vi "PicoScope3000aGetBlock.vi"(0 "error in":errorcluster, 2 "handle in":i16, 3 "Acquisition Settings":T4 {"Down Sample Ratio" min=1 step=1; "Down-Sample Mode" items=["None", "Aggregate", "Decimate", "Average"]}, 8 "Device Info":T1) -> (4 "overflow":i16, 5 "noOfSamples":u32, 6 "error out":errorcluster, 7 "handle out":i16, 9 "Buffers (Max or non-aggregated)":T3, 10 "Min Buffers":T2)   [LabVIEW 2009]
doc: "This VI collects a block of data from the oscilloscope. This can be called in a loop in order to continually collect blocks of data. The oscilloscope should first be set up by using PicoScope3000aSettings.vi. The VI outputs data arrays in two clusters (max and min). If not using aggregation, 'Min Buffers' is not used."
uses:
  ps3000a.dll
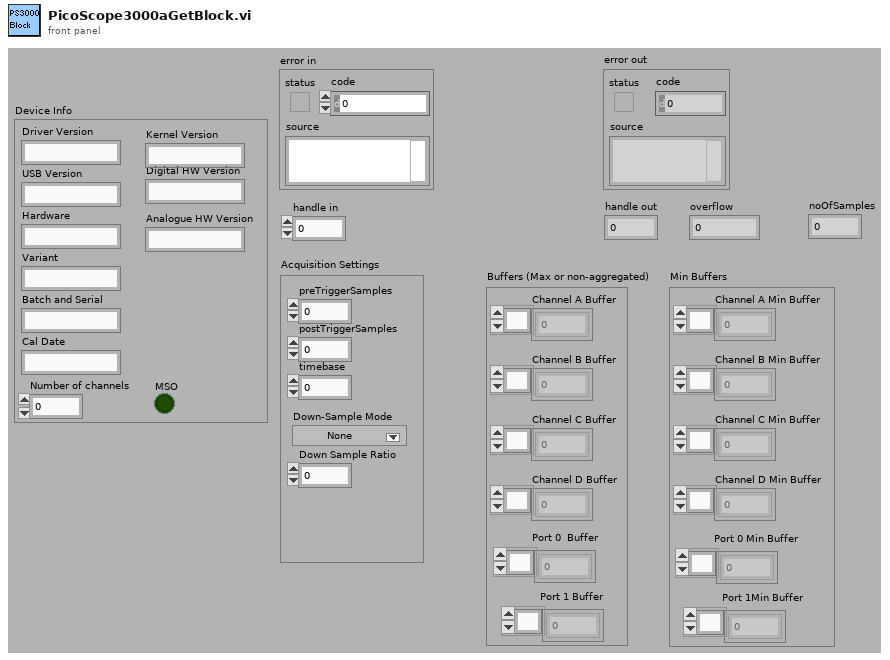
[diagram p1: front panel]
types:
  T1 = cluster{"Driver Version":string, "USB Version":string, "Hardware":string, "Variant":string, "Batch and Serial":string, "Cal Date":string, "Kernel Version":string, "Digital HW Version":string, "Analogue HW Version":string, "MSO":bool, "Number of channels":i16}
  T2 = cluster{"Channel A Min Buffer":i16[], "Channel B Min Buffer":i16[], "Channel C Min Buffer":i16[], "Channel D Min Buffer":i16[], "Port 0 Min Buffer ":i16[], "Port 1Min Buffer ":i16[]}
  T3 = cluster{"Channel D Buffer":i16[], "Channel C Buffer":i16[], "Channel B Buffer":i16[], "Channel A Buffer":i16[], "Port 0  Buffer ":i16[], "Port 1 Buffer ":i16[]}
  T4 = cluster{"preTriggerSamples":u32, "postTriggerSamples":u32, "timebase":u32, "Down-Sample Mode":i32, "Down Sample Ratio":u32}
  T5 = cluster{"Channel A Min Buffer":i16[], "Channel B Min Buffer":i16[], "Channel C Min Buffer":i16[], "Channel D Min Buffer":i16[], "Port 0 Min Buffer":i32[], "Port 1 Min Buffer":i32[]}
  T6 = cluster{"Channel D Buffer":i16[], "Channel C Buffer":i16[], "Channel B Buffer":i16[], "Channel A Buffer":i16[], "Port 0 Max Buffer":i32[], "Port 1 Max Buffer":i32[]}
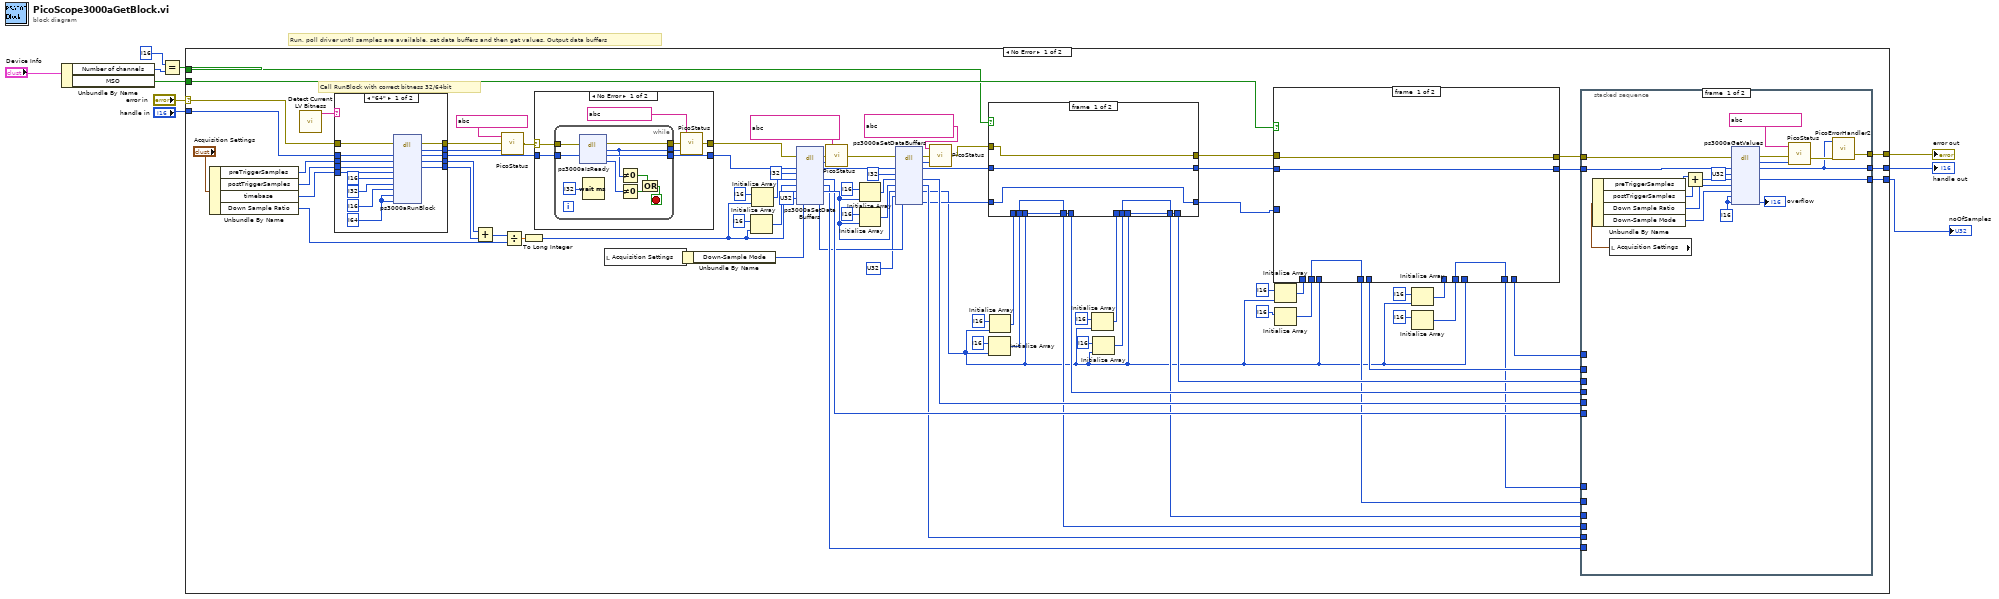
[diagram p0: block diagram]
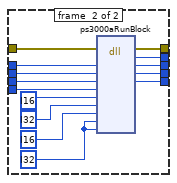
[diagram p2: hidden frame]
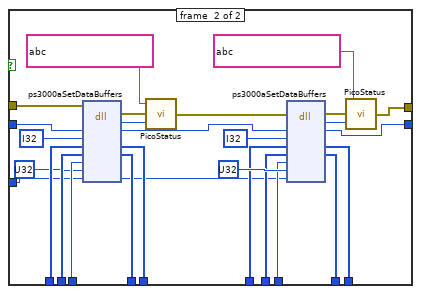
[diagram p3: hidden frame]
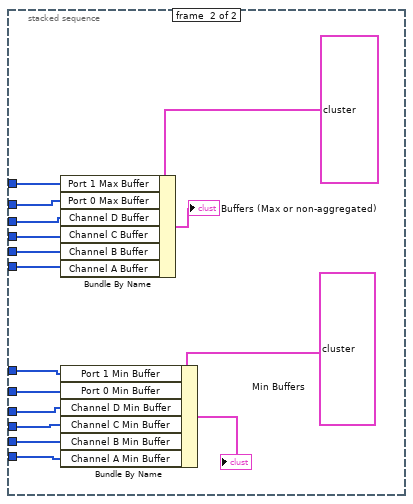
[diagram p4: hidden frame]
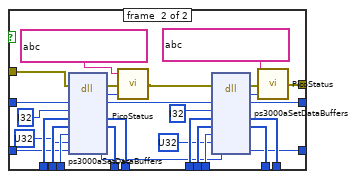
[diagram p6: hidden frame]
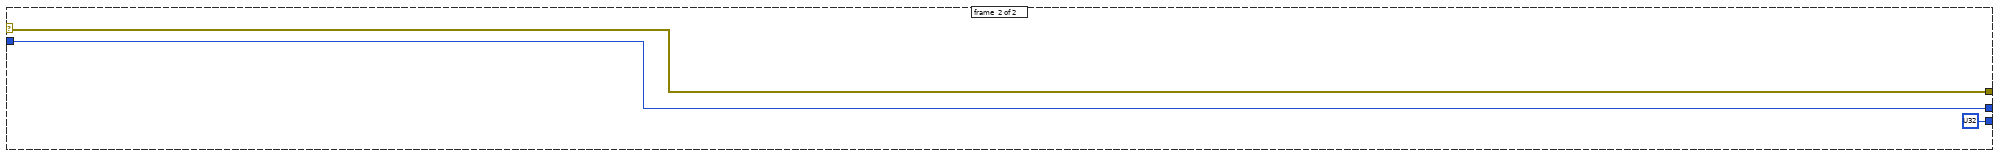
[diagram p7: hidden frame]
diagram:
  # "Run, poll driver until samples are available, set data buffers and then get values. Output data buffers"
  n1 = Unbundle By Name("Device Info") -> ("Number of channels"=w4:i16, "MSO"=w3:bool)
  n2 = Equal?(x=i16 ?, y=w4) -> (x = y?=w2:bool)
  n3 = case shown="No Error" "error in" {
    selector: "error in" -> [w64 w248]
    tunnel: [w65 w248] -> w9
    tunnel: "handle in" -> [w63 w247]
    tunnel: [w62 w247] -> w7
    tunnel: [w15 u32 ? ("noOfSamples")] -> w6
    tunnel: w3 -> [w13 _]
    tunnel: w2 -> [w12 _]
    frame #0 {
      # "Call RunBlock with correct bitness 32/64bit"
      n4 = Unbundle By Name("Acquisition Settings") -> ("preTriggerSamples"=w79:u32, "postTriggerSamples"=w78:u32, "timebase"=w80:u32, "Down Sample Ratio"=w14:u32)
      n5 = call "Detect Current LV Bitness.vi"() -> ("bitness"=w11:string)  [unwired: 11 in]
      n6 = case shown="\"64\"" w11 {
        tunnel: [w110 w124] -> w96
        tunnel: [w109 w123] -> w92
        tunnel: [w108 w122] -> w91
        tunnel: w80 -> [w107 w121]
        tunnel: w79 -> [w106 w120]
        tunnel: w78 -> [w105 w119]
        tunnel: [w104 w118] -> w77
        tunnel: [w103 w117] -> w76
        tunnel: w64 -> [w102 w116]
        tunnel: w63 -> [w101 w115]
        frame #0 {
          w97 = i64 ? ("pParameter")
          n7 = dll-call lib="ps3000a.dll" fn="ps3000aRunBlock" ("ps3000.dll:_ps3000_open_unit@0")(error in=w102, "handle"=w101, "preTriggerSamples"=w106, "postTriggerSamples"=w105, "timebase"=w107, "oversample"=i16 ?, "timeindisposed"=i32 ? ("pParameter"), "segmentIndex"=i16 ? ("pParameter"), "lpReady"=w97, "pParameter"=w97) -> (error out=w103:errorcluster, "PICO_STATUS"=w104:i32, "handle"=w110:i16, "preTriggerSamples"=w109:u32, "postTriggerSamples"=w108:u32)  [unwired: 8 in, 1 out]
        }
        frame #1 {
          w111 = i32 ? ("pParameter")
          n8 = dll-call lib="ps3000a.dll" fn="ps3000aRunBlock" ("ps3000.dll:_ps3000_open_unit@0")(error in=w116, "handle"=w115, "preTriggerSamples"=w120, "postTriggerSamples"=w119, "timebase"=w121, "oversample"=i16 ?, "timeindisposed"=i32 ? ("pParameter"), "segmentIndex"=i16 ? ("pParameter"), "lpReady"=w111, "pParameter"=w111) -> (error out=w117:errorcluster, "PICO_STATUS"=w118:i32, "handle"=w124:i16, "preTriggerSamples"=w123:u32, "postTriggerSamples"=w122:u32)  [unwired: 8 in, 1 out]
        }
      }
      n9 = Add(x=w92, y=w91) -> (x+y=w42:u32)
      n10 = call "PicoStatus.vi"("PICO STATUS"=w77, "error in"=w76, "source"=string ?) -> ("error out"=w75:errorcluster)
      n11 = Divide(x=w42, y=w14) -> (x/y=w41:dbl)
      n12 = To Long Integer(number=w41) -> (32bit integer=w40:i32)
      n13 = case shown="No Error" w75 {
        selector: w75 -> [w195 w208]
        tunnel: w96 -> [w197 w209]
        tunnel: [w196 w209] -> w95
        tunnel: [w194 w208] -> w83
        frame #0 {
          n14 = while {
            tunnel: [w207] -> w196
            tunnel: w197 -> [w206]
            tunnel: [w201] -> w192
            tunnel: w195 -> [w200]
            tunnel: [w199] -> w193
            stop <- w205 stop-if-true
            n15 = dll-call lib="ps3000a.dll" fn="ps3000aIsReady" ("ps3000.dll:_ps3000_open_unit@0")(error in=w200, "handle"=w206) -> (error out=w199:errorcluster, "status"=w201:i32, "handle"=w207:i16, "ready"=w202:i16)  [unwired: 3 in, 1 out]
            n16 = Wait (ms)(milliseconds to wait=i32 ?) -> ()  [unwired: 1 out]
            n17 = Not Equal To 0?(x=w201) -> (x != 0?=w203:bool)
            n18 = Not Equal To 0?(x=w202) -> (x != 0?=w204:bool)
            n19 = Or(x=w203, y=w204) -> (x .or. y?=w205:bool)
          }
          n20 = call "PicoStatus.vi"("PICO STATUS"=w192, "error in"=w193, "source"=string ?) -> ("error out"=w194:errorcluster)
        }
        frame #1 {
        }
      }
      n21 = local read "Acquisition Settings"() -> (w39:T4)
      n22 = Unbundle By Name(w39) -> ("Down-Sample Mode"=w37:i32)
      n23 = Initialize Array(i16 ? ("element"), w40) -> (w60:i16[])
      n24 = Initialize Array(i16 ? ("element"), w40) -> (w90:i16[])
      n25 = dll-call lib="ps3000a.dll" fn="ps3000aSetDataBuffers" ("ps3000.dll:_ps3000_open_unit@0")(error in=w83, "handle"=w95, "channel"=i32 ?, "bufferMax"=w90, "bufferMin"=w60, "bufferLth"=w40, "segmentIndex"=u32 ?, "mode"=w37) -> (error out=w73:errorcluster, "PICO_STATUS"=w74:i32, "handle"=w94:i16, "bufferMax"=w47:i16[], "bufferMin"=w43:i16[], "bufferLth"=w51:i32, "mode"=w36:i32)  [unwired: 4 in, 1 out]
      n26 = call "PicoStatus.vi"("PICO STATUS"=w74, "error in"=w73, "source"=string ?) -> ("error out"=w72:errorcluster)
      n27 = Initialize Array(i16 ? ("element"), w51) -> (w87:i16[])
      n28 = Initialize Array(i16 ? ("element"), w51) -> (w58:i16[])
      n29 = dll-call lib="ps3000a.dll" fn="ps3000aSetDataBuffers" ("ps3000.dll:_ps3000_open_unit@0")(error in=w72, "handle"=w94, "channel"=i32 ?, "bufferMax"=w87, "bufferMin"=w58, "bufferLth"=w51, "segmentIndex"=u32 ?, "mode"=w36) -> (error out=w70:errorcluster, "PICO_STATUS"=w71:i32, "handle"=w93:i16, "bufferMax"=w48:i16[], "bufferMin"=w44:i16[], "bufferLth"=w16:i32, "mode"=w35:i32)  [unwired: 4 in, 1 out]
      n30 = call "PicoStatus.vi"("PICO STATUS"=w71, "error in"=w70, "source"=string ?) -> ("error out"=w69:errorcluster)
      n31 = Initialize Array(i16 ? ("element"), w16) -> (w55:i16[])
      n32 = Initialize Array(i16 ? ("element"), w16) -> (w86:i16[])
      n33 = Initialize Array(i16 ? ("element"), w16) -> (w85:i16[])
      n34 = Initialize Array(i16 ? ("element"), w16) -> (w52:i16[])
      n35 = case shown="True" w12 {
        tunnel: w93 -> [w214 w245]
        tunnel: [w214 w243] -> w24
        tunnel: w86 -> [w216 w242]
        tunnel: w85 -> [w215 w241]
        tunnel: [w215 w240] -> w50
        tunnel: [w216 w239] -> w49
        tunnel: w69 -> [w213 w236]
        tunnel: [w213 w230] -> w25
        tunnel: w55 -> [w212 w227]
        tunnel: w52 -> [w211 w226]
        tunnel: [w211 w225] -> w46
        tunnel: [w212 w224] -> w45
        tunnel: w16 -> [_ w223]
        tunnel: w16 -> [_ w222]
        tunnel: w35 -> [w210 w221]
        tunnel: [w210 w217] -> w21
        frame #0 {
        }
        frame #1 {
          n36 = dll-call lib="ps3000a.dll" fn="ps3000aSetDataBuffers" ("ps3000.dll:_ps3000_open_unit@0")(error in=w236, "handle"=w245, "channel"=i32 ?, "bufferMax"=w242, "bufferMin"=w227, "bufferLth"=w223, "segmentIndex"=u32 ?, "mode"=w221) -> (error out=w234:errorcluster, "PICO_STATUS"=w235:i32, "handle"=w244:i16, "bufferMax"=w239:i16[], "bufferMin"=w224:i16[], "mode"=w220:i32)  [unwired: 5 in, 1 out]
          n37 = call "PicoStatus.vi"("PICO STATUS"=w235, "error in"=w234, "source"=string ?) -> ("error out"=w233:errorcluster)
          n38 = dll-call lib="ps3000a.dll" fn="ps3000aSetDataBuffers" ("ps3000.dll:_ps3000_open_unit@0")(error in=w233, "handle"=w244, "channel"=i32 ?, "bufferMax"=w241, "bufferMin"=w226, "bufferLth"=w222, "segmentIndex"=u32 ?, "mode"=w220) -> (error out=w231:errorcluster, "PICO_STATUS"=w232:i32, "handle"=w243:i16, "bufferMax"=w240:i16[], "bufferMin"=w225:i16[], "mode"=w217:i32)  [unwired: 5 in, 1 out]
          n39 = call "PicoStatus.vi"("PICO STATUS"=w232, "error in"=w231, "source"=string ?) -> ("error out"=w230:errorcluster)
        }
      }
      n40 = Initialize Array(i16 ? ("element"), w16) -> (w31:i16[])
      n41 = Initialize Array(i16 ? ("element")) -> (w30:i16[])  [unwired: 1 in]
      n42 = Initialize Array(i16 ? ("element"), w16) -> (w26:i16[])
      n43 = Initialize Array(i16 ? ("element")) -> (w27:i16[])  [unwired: 1 in]
      n44 = case shown="True" w13 {
        tunnel: w25 -> [w126 w156]
        tunnel: w24 -> [w125 w155]
        tunnel: w31 -> [_ w153]
        tunnel: w30 -> [w128 w152]
        tunnel: w16 -> [_ w151]
        tunnel: w16 -> [_ w145]
        tunnel: w27 -> [w127 w146]
        tunnel: w26 -> [_ w147]
        tunnel: [w128 w144] -> w17
        tunnel: [_ w143] -> w19
        tunnel: [w127 w142] -> w18
        tunnel: [_ w141] -> w20
        tunnel: [w125 w135] -> w22
        tunnel: [w126 w134] -> w23
        tunnel: w21 -> [_ w132]
        frame #0 {
        }
        frame #1 {
          n45 = dll-call lib="ps3000a.dll" fn="ps3000aSetDataBuffers" ("ps3000.dll:_ps3000_open_unit@0")(error in=w156, "handle"=w155, "channel"=i32 ?, "bufferMax"=w153, "bufferMin"=w152, "bufferLth"=w151, "segmentIndex"=u32 ?, "mode"=w132) -> (error out=w139:errorcluster, "PICO_STATUS"=w140:i32, "handle"=w133:i16, "bufferMax"=w143:i16[], "bufferMin"=w144:i16[], "mode"=w131:i32)  [unwired: 5 in, 1 out]
          n46 = call "PicoStatus.vi"("PICO STATUS"=w140, "error in"=w139, "source"=string ?) -> ("error out"=w136:errorcluster)
          n47 = dll-call lib="ps3000a.dll" fn="ps3000aSetDataBuffers" ("ps3000.dll:_ps3000_open_unit@0")(error in=w136, "handle"=w133, "channel"=i32 ?, "bufferMax"=w147, "bufferMin"=w146, "bufferLth"=w145, "segmentIndex"=u32 ?, "mode"=w131) -> (error out=w137:errorcluster, "PICO_STATUS"=w138:i32, "handle"=w135:i16, "bufferMax"=w141:i16[], "bufferMin"=w142:i16[])  [unwired: 6 in, 1 out]
          n48 = call "PicoStatus.vi"("PICO STATUS"=w138, "error in"=w137, "source"=string ?) -> ("error out"=w134:errorcluster)
        }
      }
      n49 = stacked-sequence {
        tunnel: w22 -> [w174 _]
        tunnel: [w168 _] -> w65
        tunnel: [w157 _] -> w62
        tunnel: w50 -> [_ w180]
        tunnel: w49 -> [_ w181]
        tunnel: w48 -> [_ w182]
        tunnel: w47 -> [_ w179]
        tunnel: w46 -> [_ w186]
        tunnel: w45 -> [_ w185]
        tunnel: w44 -> [_ w184]
        tunnel: w43 -> [_ w183]
        tunnel: w23 -> [w160 _]
        tunnel: w20 -> [_ w178]
        tunnel: w19 -> [_ w177]
        tunnel: w18 -> [_ w176]
        tunnel: w17 -> [_ w175]
        tunnel: [w159 _] -> w15
        frame #0 {
          w172 = i16 ? ("overflow")
          n50 = local read "Acquisition Settings"() -> (w166:T4)
          n51 = Unbundle By Name(w166) -> ("preTriggerSamples"=w163:u32, "postTriggerSamples"=w164:u32, "Down Sample Ratio"=w165:u32, "Down-Sample Mode"=w161:i32)
          n52 = Add(x=w163, y=w164) -> (x+y=w162:u32)
          n53 = dll-call lib="ps3000a.dll" fn="ps3000aGetValues" ("ps3000.dll:_ps3000_open_unit@0")(error in=w160, "handle"=w174, "startIndex"=u32 ?, "noOfSamples"=w162, "downSampleRatio"=w165, "downSampleRatioMode"=w161, "segmentIndex"=w172, "overflow"=w172) -> (error out=w171:errorcluster, "PICO_STATUS"=w158:i32, "handle"=w157:i16, "noOfSamples"=w159:u32, "overflow"=→"overflow":i16)  [unwired: 6 in, 1 out]
          n54 = call "PicoStatus.vi"("PICO STATUS"=w158, "error in"=w171, "source"=string ?) -> ("error out"=w169:errorcluster)
          n55 = call "PicoErrorHandler2.vi"("error in (no error)"=w169, "handle In"=w157) -> ("error out"=w168:errorcluster)  [unwired: 9 in]
        }
        frame #1 {
          n56 = Bundle By Name(cluster=T6 ? ("Buffers (Max or non-aggregated)"), "Port 1 Max Buffer"=w178, "Port 0 Max Buffer"=w177, "Channel D Buffer"=w180, "Channel C Buffer"=w181, "Channel B Buffer"=w182, "Channel A Buffer"=w179) -> (→"Buffers (Max or non-aggregated)":T6)
          n57 = Bundle By Name(cluster=T5 ? ("Min Buffers"), "Port 1 Min Buffer"=w176, "Port 0 Min Buffer"=w175, "Channel D Min Buffer"=w186, "Channel C Min Buffer"=w185, "Channel B Min Buffer"=w184, "Channel A Min Buffer"=w183) -> (→"Min Buffers":T5)
        }
      }
    }
    frame #1 {
    }
  }
  "error out" <- w9
  "handle out" <- w7
  "noOfSamples" <- w6
